vi "Vision Research Phantom Series PhCon PhGetVisibleIp.vi"(5 "Error In (no error)":errorcluster) -> (16 "pCnt":u32, 17 "pIpAddress":u32[](array[numeric]), 19 "Error Out":errorcluster)   [LabVIEW 2013, in "VRI.lvlib"]
doc: "PhCon.dll\n\nPhGetVisibleIp\nHRESULT PhGetVisibleIp(PUINT pCnt, PUINT pIpAddress);\n\nParameters Description\npCnt (out) Count of visible camera IP addresses.\npIpAddress (out) Array of visible camera IP addresses.\nReturn HRESULT (0 = Ok)\nComments Use the function to obtain an array of the IP addresses\n of all the cameras in the visible, or \"Connect Only To\"\n list. The visible list contains the cameras you wish to be\n connected to, no matter if they are or not on the network\n of your computer at that moment.\n\n If the visible list contains at least one camera, the UDP\n broadcast mechanism used to detect cameras is not\n proceeded with. The computer connects only to cameras\n in the visible list and does not connect to cameras in the\n ignored list.\n \n If you include a camera in both the visible and ignored\n lists, the visible list will have priority so the camera will \n be connected to your computer."
uses:
  VRI.lvlib
  Phantom DLLs/PhCon.dll
panel:
  # "For instructions on the use of this VI, press Ctrl+H to display the help window and move the mouse over the icon, controls, and indicators"
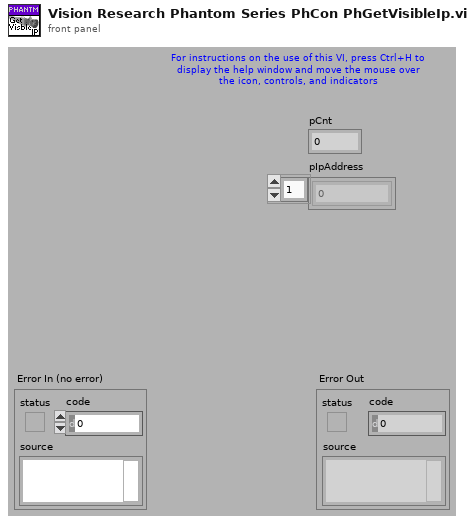
[diagram p1: front panel]
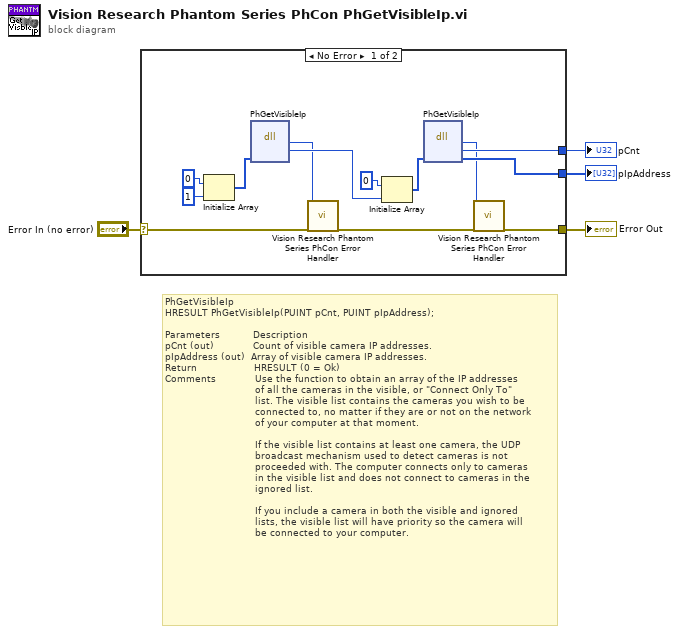
[diagram p0: block diagram]
diagram:
  # "PhGetVisibleIp\nHRESULT PhGetVisibleIp(PUINT pCnt, PUINT pIpAddress);\n\nParameters           Description\npCnt (out)             Count of visible camera IP addresses.\npIpAddress (out)  Array of visible camera IP addresses.\nReturn                   HRESULT (0 = Ok)\nComments             Use the function to obtain an array of the IP addresses\n                              of all the cameras in the visible, or \"Connect Only To\"\n                              list. The visible list contains the cameras you wish to be\n                              connected to, no matter if they are or not on the network\n                              of your computer at that moment.\n\n                              If the visible list contains at least one camera, the UDP\n                              broadcast mechanism used to detect cameras is not\n                              proceeded with. The computer connects only to cameras\n                              in the visible list and does not connect to cameras in the\n                              ignored list.\n \n                              If you include a camera in both the visible and ignored\n                              lists, the visible list will have priority so the camera will \n                              be connected to your computer."
  n1 = case shown="No Error" "Error In (no error)" {
    selector: "Error In (no error)" -> [w17 w18]
    tunnel: [w16 w18] -> w3
    tunnel: [w15 _] -> w2
    tunnel: [w14 _] -> w1
    frame No Error {
      n2 = Initialize Array(u32 0 ("element"), 1 ("dimension size")) -> (w6:u32[])
      n3 = dll-call lib="C:/Projects/SDK/32-bit/Vision Research Phantom Series Labview Driver/Phantom DLLs/PhCon.dll" fn="PhGetVisibleIp"("pIpAddress"=w6) -> ("HRESULT"=w8:i32, "pCnt"=w10:u32)  [unwired: 3 in, 4 out]
      n4 = call "Vision Research Phantom Series PhCon Error Handler.vi"("ErrNo"=w8, "Error In (no error)"=w17) -> ("Error Out"=w9:errorcluster)  [unwired: 17 out]
      n5 = Initialize Array(u32 0 ("element"), w10) -> (w11:u32[])
      n6 = dll-call lib="C:/Projects/SDK/32-bit/Vision Research Phantom Series Labview Driver/Phantom DLLs/PhCon.dll" fn="PhGetVisibleIp"("pIpAddress"=w11) -> ("HRESULT"=w13:i32, "pCnt"=w15:u32, "pIpAddress"=w14:u32[])  [unwired: 3 in, 3 out]
      n7 = call "Vision Research Phantom Series PhCon Error Handler.vi"("ErrNo"=w13, "Error In (no error)"=w9) -> ("Error Out"=w16:errorcluster)  [unwired: 17 out]
    }
    frame Error {
    }
  }
  "Error Out" <- w3
  "pIpAddress" <- w1
  "pCnt" <- w2
